vi "Teleop.vi"(10 "Match Info":T2={"Autonomous Elapsed Seconds"=0.0, "TeleOp Elapsed Seconds"=0.0, "Disabled Elapsed Seconds"=0.0, "Visited Autonomous"=FALSE, "Visited TeleOp"=FALSE, "Visited Disabled"=FALSE, "Autonomous Settings"={"Autonomous Style"=enum."Independent", "VI Refnum"=refnum}}, 11 "Call Context":T3) -> ()   [LabVIEW 2017]
doc: "This VI is called for each TeleOp packet received from the DS where the robot is not disabled. It is often used to read from the joysticks and update I/O or to update setpoints for timed control loops. It should complete and return within 20 milliseconds or it may miss DS packets."
uses:
  <vilib>/Rock Robotics/WPI/DriverStation/WPI_DriverStationDerivedRobotMode.ctl
  <vilib>/Rock Robotics/WPI/DriverStation/WPI_DriverStationMatch Info.ctl
  C:/Users/Public/Documents/Cross The Road Electronics/Phoenix-LabVIEW/Motor Controller/Controls/CTRE_Phoenix_MotorControl_FeedbackDevice.ctl
  C:/Users/Public/Documents/Cross The Road Electronics/Phoenix-LabVIEW/Motor Controller/Controls/CTRE_Phoenix_MotorControl_ControlMode.ctl
  <vilib>/Rock Robotics/WPI/Utilities/WPI_GetSetVariantRefNum.vi
  C:/Users/Public/Documents/Cross The Road Electronics/Phoenix-LabVIEW/Motor Controller/Get/CTRE_Phoenix_MotorController_GetVoltage.vi
  C:/Users/Public/Documents/Cross The Road Electronics/Phoenix-LabVIEW/Motor Controller/Get/CTRE_Phoenix_MotorController_GetSelectedSensorData.vi
panel:
  out "SensorPosRotations":i32
  out "Motor output Plot":cluster{"Applied Throttle":dbl}(graph)
  out "Target RPM":dbl
  out "SensorRPM Velocity RPM":i32
  in  "I Zone":dbl
  in  "F":dbl
  in  "D":dbl
  in  "I":dbl
  in  "P":dbl
  out "Applied Output":dbl
  out "Speed Closed Loop Plots":T1(graph)
  # "Use the Left Y-axis on Logitech Gamepad.\n\nVelocityNativeUnits = Change In Sensor / 100mS\nalso\nVelocityNativeUnits = RPM / 600 * SensorUnitsPerRotation\n\nFgain = 100% X 1023 / VelocityNativeUnits , \n       where VelocityNativeUnits  is measured at 100% throttle\n\nMag Encoder has 4096 units per rotation.\n\nExample: VelocityRPM is 10198 at 100% throttle\n                 => VelocityNativeUnits = (10198 / 600 * 4096) = 69618\n                 => Fgain = (1023 / 69618)  = 0.01469"
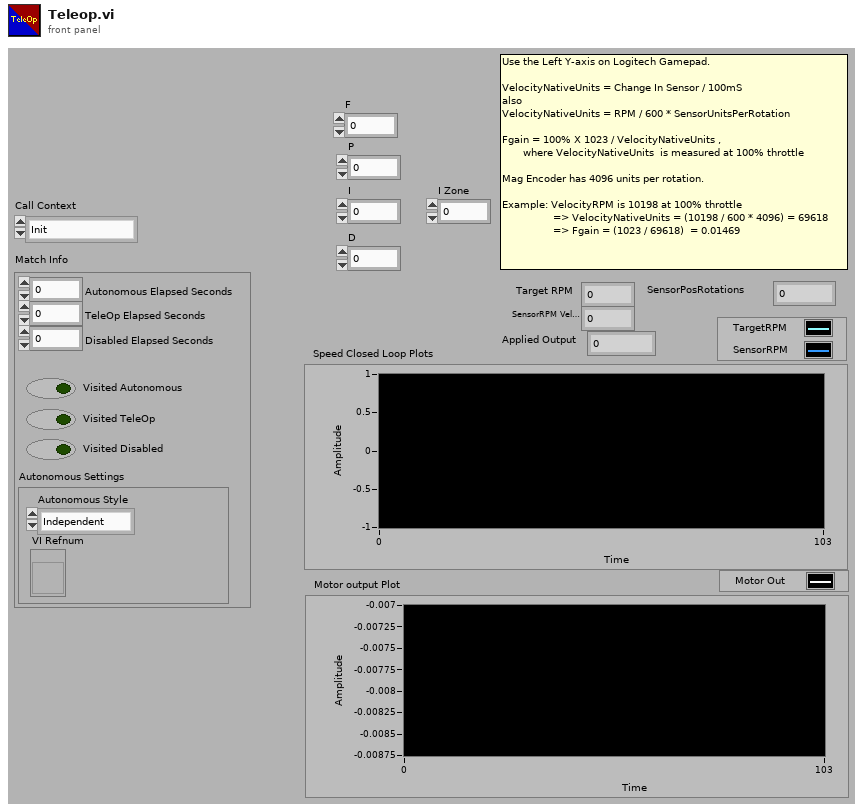
[diagram p1: front panel]
types:
  T1 = cluster{"x":dbl, "Velocity (Raw Sensor Units per 100 ms)":i32}
  T2 = typedef "WPI_DriverStationMatch Info.ctl" = cluster{"Autonomous Elapsed Seconds":dbl, "TeleOp Elapsed Seconds":dbl, "Disabled Elapsed Seconds":dbl, "Visited Autonomous":bool, "Visited TeleOp":bool, "Visited Disabled":bool, "Autonomous Settings":cluster{"Autonomous Style":enum16{"Iterative", "Independent"}, "VI Refnum":refnum<vi>}}
  T3 = typedef "WPI_DriverStationDerivedRobotMode.ctl" = enum16{"Init", "Execute", "Stop"}
  T4 = typedef "CTRE_Phoenix_MotorControl_FeedbackDevice.ctl" = i8
  T5 = typedef "WPI_MotorControlDeviceRef.ctl" = cluster{"DeviceStatus":errorcluster, "Type":T6, "PWM":cluster{"PWM Channel":T7, "DeadBand":T8}, "CAN":cluster{"Device Number":u8, "SetOutput VI Ref":variant, "GetOutput VI Ref":variant, "Enable VI Ref":variant, "Disable VI Ref":variant, "Data":variant}, "Invert":bool, "DIO PWM":cluster{"PWM \"Enable\" Channel":T7, "DIOChannel":T9, "PWM Rate":dbl}}
  T6 = typedef "WPI_MotorControlType.ctl" = enum16{"PWM", "CAN", "DIO PWM"}
  T7 = typedef "FPGA_DIOPWMChannel.ctl" = enum8{"PWM 0", "PWM 1", "PWM 2", "PWM 3", "PWM 4", "PWM 5", "PWM 6", "PWM 7", "PWM 8", "PWM 9", "PWM MXP 0", "PWM MXP 1", "PWM MXP 2", "PWM MXP 3", "PWM MXP 4", "PWM MXP 5", "PWM MXP 6", "PWM MXP 7", "PWM MXP 8", "PWM MXP 9", "Invalid"}
  T8 = typedef "WPI_PWMDeadband.ctl" = cluster{"Name":string, "maxPositivePwm":i32, "minPositivePwm":i32, "centerPwm":i32, "maxNegativePwm":i32, "minNegativePwm":i32, "angularRange":u16}
  T9 = typedef "FPGA_DIOChannel.ctl" = enum8{"DIO 0", "DIO 1", "DIO 2", "DIO 3", "DIO 4", "DIO 5", "DIO 6", "DIO 7", "DIO 8", "DIO 9", "DIO MXP 0", "DIO MXP 1", "DIO MXP 2", "DIO MXP 3", "DIO MXP 4", "DIO MXP 5", "DIO MXP 6", "DIO MXP 7", "DIO MXP 8", "DIO MXP 9", "DIO MXP 10", "DIO MXP 11", "DIO MXP 12", "DIO MXP 13", "DIO MXP 14", "DIO MXP 15", "SPI Port CS1", "SPI Port CS2", "SPI Port CS3", "SPI Port MISO", "SPI Port MOSI", "Invalid"}
  T10 = typedef "WPI_JoystickDevRef.ctl" = cluster{"Device":T11}
  T11 = typedef "WPI_JoystickDeviceEnum.ctl" = enum16{"USB 0", "USB 1", "USB 2", "USB 3", "USB 4", "USB 5"}
  T12 = typedef "CTRE_Phoenix_MotorControl_ControlMode.ctl" = u16
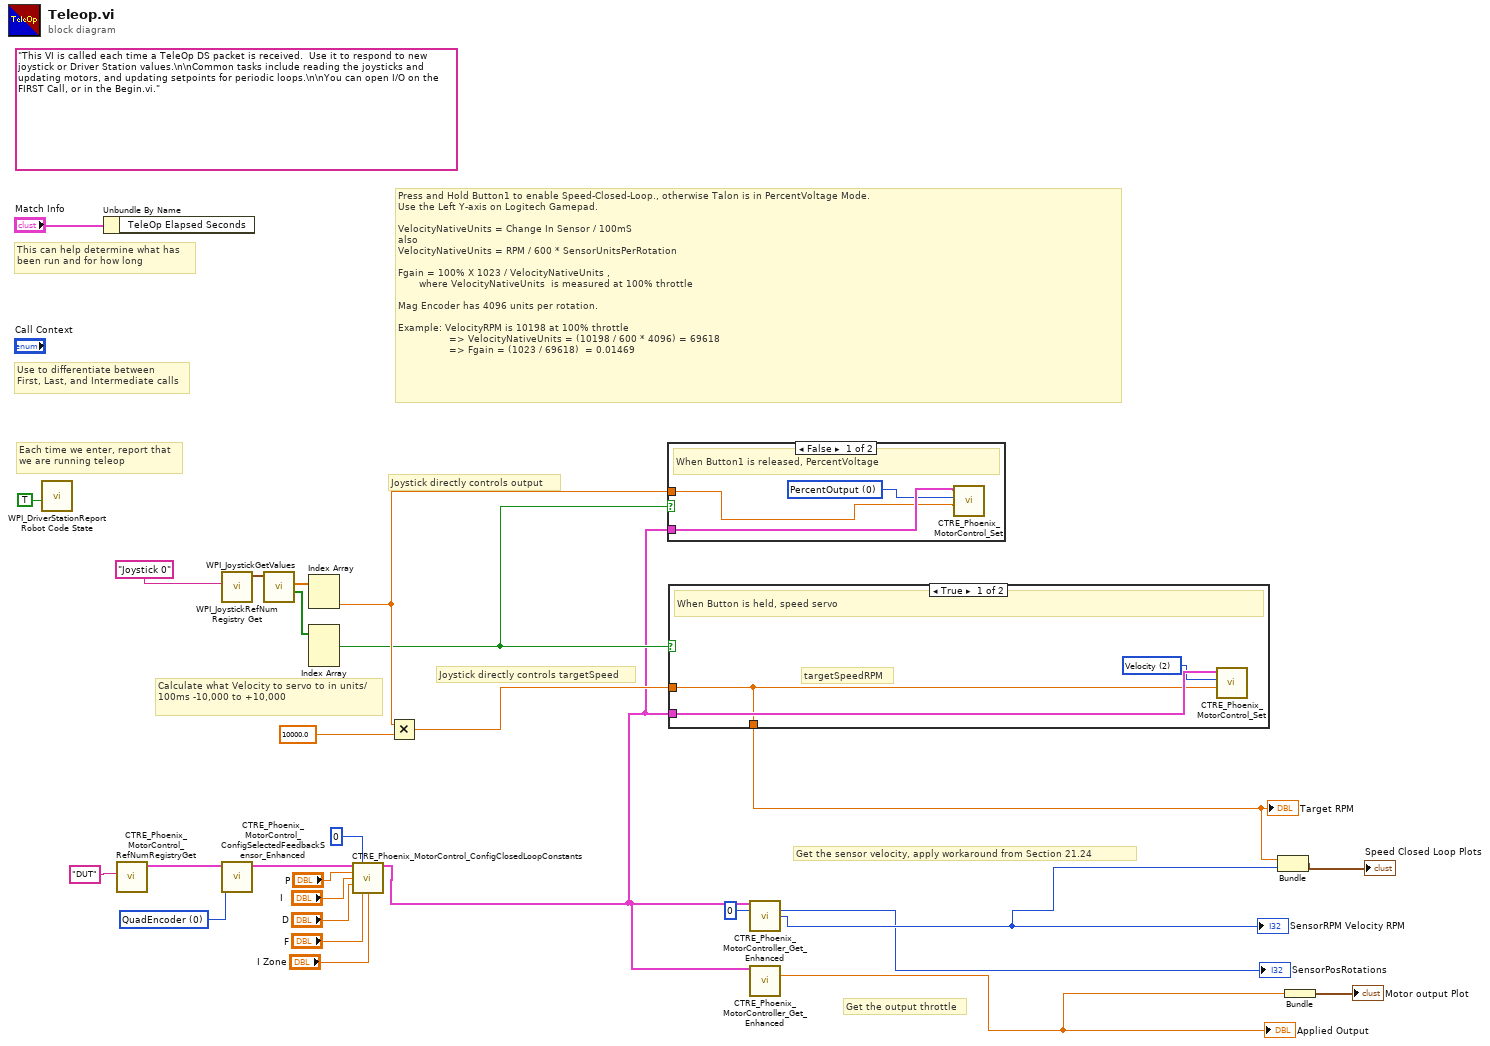
[diagram p0: block diagram]
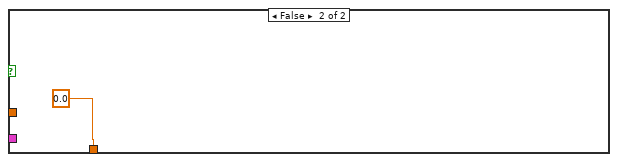
[diagram p3: hidden frame]
diagram:
  w1 = T4 0 items=["None"=-1, "QuadEncoder"=0, "Analog"=2, "Tachometer"=4, "Pulse Width Encoded Position"=8, "Sensor Sum (S0 + S1)"=9, "Sensor Difference (D0 - D1)"=10, "Remote Source 0"=11, "Remote Source 1"=12, "Software Emulated"=15] ("Feedback Device")
  (unwired) "This VI is called each time a TeleOp DS packet is received.  Use it to respond to new joystick or Driver Station values.\n\nCommon tasks include reading the joysticks and updating motors, and updating setpoints for periodic loops.\n\nYou can open I/O on the FIRST Call, or in the Begin.vi."
  # "Press and Hold Button1 to enable Speed-Closed-Loop., otherwise Talon is in PercentVoltage Mode.  \nUse the Left Y-axis on Logitech Gamepad.\n\nVelocityNativeUnits = Change In Sensor / 100mS\nalso\nVelocityNativeUnits = RPM / 600 * SensorUnitsPerRotation\n\nFgain = 100% X 1023 / VelocityNativeUnits , \n       where VelocityNativeUnits  is measured at 100% throttle\n\nMag Encoder has 4096 units per rotation.\n\nExample: VelocityRPM is 10198 at 100% throttle\n                 => VelocityNativeUnits = (10198 / 600 * 4096) = 69618\n                 => Fgain = (1023 / 69618)  = 0.01469"
  # "Get the output throttle"
  # "Get the sensor velocity, apply workaround from Section 21.24"
  # "Joystick directly controls targetSpeed"
  # "Joystick directly controls output"
  # "Calculate what Velocity to servo to in units/100ms -10,000 to +10,000"
  # "Each time we enter, report that\nwe are running teleop"
  # "Use to differentiate between\nFirst, Last, and Intermediate calls"
  # "This can help determine what has\nbeen run and for how long"
  n1 = call <vilib>:"WPI_DriverStationReport Robot Code State.vi"("TeleOp"=TRUE ("Autonomous")) -> ()  [unwired: 10 in, 1 out]
  n2 = Unbundle By Name("Match Info") -> ()  [unwired: 1 out]
  n3 = call "CTRE_Phoenix_MotorControl_RefNumRegistryGet.vi"("refnum name"="DUT") -> ("PhoenixMotorControlDevRef"=w13:T5)  [unwired: 9 in, 1 out]
  n4 = call <vilib>:"WPI_JoystickRefNum Registry Get.vi"("refnum name"="Joystick 0") -> ("JoystickDevRef"=w26:T10)  [unwired: 1 in, 9 out]
  n5 = call "CTRE_Phoenix_MotorControl_ConfigSelectedFeedbackSensor_Enhanced.vi"("Feedback Device"=w1, "PhoenixMotorControlDevRef"=w13) -> ("PhoenixMotorControlDevRef"=w14:T5)  [unwired: 8 in, 1 out]
  n6 = call <vilib>:"WPI_JoystickGetValues.vi"("JoystickDevRef"=w26) -> ("Buttons"=w23:bool[], "Axes"=w24:dbl[])  [unwired: 6 in, 3 out]
  n7 = Index Array(array=w24) -> (element #2=w22:dbl)  [unwired: 2 in, 1 out]
  n8 = Index Array(array=w23) -> (element #1=w20:bool)  [unwired: 3 in, 2 out]
  n9 = call "CTRE_Phoenix_MotorControl_ConfigClosedLoopConstants.vi"("PhoenixMotorControlDevRef"=w14, "slotIdx"=0, "P"="P", "I"="I", "D"="D", "F"="F", "I Zone"="I Zone") -> ("PhoenixMotorControlDevRef"=w4:T5)  [unwired: 7 in, 1 out]
  n10 = Multiply(x=w22, y=10000.0) -> (x*y=w17:dbl)
  n11 = case shown="False" w20 {
    tunnel: w22 -> [w30 _]
    tunnel: w4 -> [w31 _]
    frame False {
      w29 = T12 0 items=["PercentOutput"=0, "Position"=1, "Velocity"=2, "Follower"=5, "MotionProfile"=6, "MotionMagic"=7, "MotionMagicArc"=8, "TimedPercentOutput"=9, "Disabled"=15] ("Control Mode")
      # "When Button1 is released, PercentVoltage"
      n12 = call "CTRE_Phoenix_MotorControl_Set.vi"("Output"=w30, "Control Mode"=w29, "PhoenixMotorControlDevRef"=w31) -> ()  [unwired: 7 in, 2 out]
    }
    frame True {
    }
  }
  n13 = case shown="True" w20 {
    tunnel: w17 -> [w33 _]
    tunnel: w4 -> [w34 _]
    tunnel: [w33 0.0 ("x")] -> w16
    frame True {
      w32 = T12 2 items=["PercentOutput"=0, "Position"=1, "Velocity"=2, "Follower"=5, "MotionProfile"=6, "MotionMagic"=7, "MotionMagicArc"=8, "TimedPercentOutput"=9, "Disabled"=15] ("Control Mode")
      # "targetSpeedRPM"
      # "When Button is held, speed servo"
      n14 = call "CTRE_Phoenix_MotorControl_Set.vi"("Output"=w33, "Control Mode"=w32, "PhoenixMotorControlDevRef"=w34) -> ()  [unwired: 7 in, 2 out]
    }
    frame False {
    }
  }
  "Target RPM" <- w16
  n15 = call-poly "CTRE_Phoenix_MotorController_Get_Enhanced.vi"("PhoenixMotorControlDevRef"=w4, "pidLoopIdx"=u32 0) -> ("Position (Raw Sensor Units)"=→"SensorPosRotations":i32, "Velocity (Raw Sensor Units per 100 ms)"=w7:i32)  [unwired: 10 in, 2 out]
  "SensorRPM Velocity RPM" <- w7
  n16 = call-poly "CTRE_Phoenix_MotorController_Get_Enhanced.vi"("PhoenixMotorControlDevRef"=w4) -> ("Percent Output"=w5:dbl)  [unwired: 10 in, 4 out]
  "Applied Output" <- w5
  n17 = Bundle("x"=w16, "Velocity (Raw Sensor Units per 100 ms)"=w7) -> (→"Speed Closed Loop Plots":T1)  [unwired: 1 in]
  n18 = Bundle("Percent Output"=w5) -> (→"Motor output Plot":cluster{"Percent Output":dbl})  [unwired: 1 in]
